vi "Add Unique Anchor to Array.vi"(5 "Anchor.lvclass":refnum<class "Anchor.lvclass">, 7 "Is Unique?":bool, 9 "Input Anchor Array":refnum<class "Anchor.lvclass">[](array[class])) -> (6 "Output Anchor Array":refnum<class "Anchor.lvclass">[](array[class]))   [LabVIEW 2014]
uses:
  Anchor.lvclass
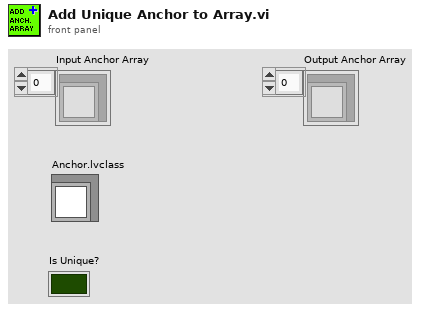
[diagram p1: front panel]
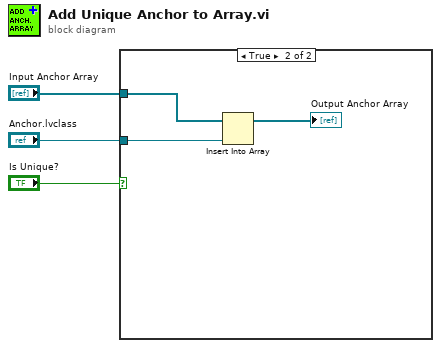
[diagram p0: block diagram]
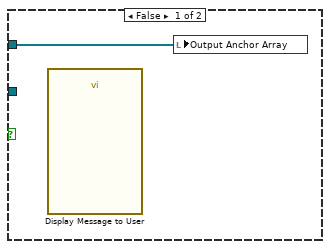
[diagram p2: hidden frame]
diagram:
  n1 = case shown="True" "Is Unique?" {
    tunnel: "Anchor.lvclass" -> [_ w6]
    tunnel: "Input Anchor Array" -> [w4 w7]
    frame False {
      n2 = call "Display Message to User"() -> ()  [unwired: 10 in, 2 out]
      n3 = local write "Output Anchor Array"(w4) -> ()
    }
    frame True {
      n4 = Insert Into Array(array=w7, new element=w6) -> (→"Output Anchor Array":refnum<class "Anchor.lvclass">[])  [unwired: 1 in]
    }
  }
